vi "Framework.Get Hardware Info.vi"(11 "Framework in":refnum<class "Framework.lvclass">) -> (2 "Hardware Info":refnum<class "Hardware Info.lvclass">, 3 "Framework out":refnum<class "Framework.lvclass">)   [LabVIEW 2017, in "DSF Core.lvlib" / "Framework.lvclass"]
uses:
  Framework.lvclass
  Hardware/Hardware Info.lvclass
  Framework.lvclass/Framework.ctl
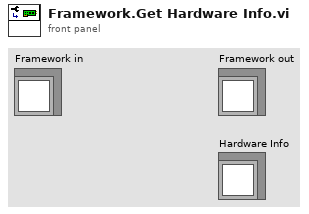
[diagram p1: front panel]
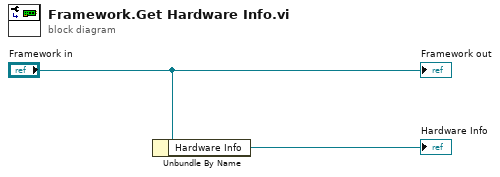
[diagram p0: block diagram]
diagram:
  n1 = Unbundle By Name("Framework in") -> ("Hardware Info"=→"Hardware Info":refnum<class "Hardware Info.lvclass">)
  "Framework out" <- "Framework in"
